vi "PeriodicFilter-Format Normal Info String.vi"(10 "Time Format String":string="%<%H:%M:%S%3u>T", 11 "Removed Info":T1[](array[typedef])) -> (3 "Array":string[](array[string]))   [LabVIEW 2017, in "Communicable State Machine.lvlib"]
uses:
  Communicable State Machine.lvlib
  Periodic String Filter Info.ctl
  _Shared/CSM Shared.lvlib
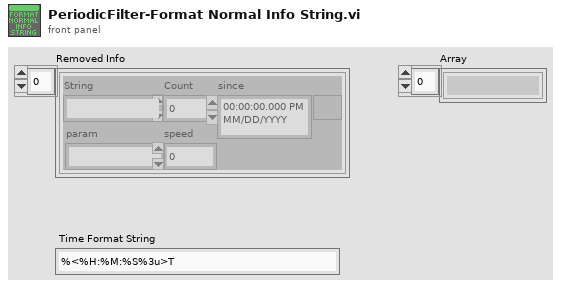
[diagram p1: front panel]
types:
  T1 = typedef "Communicable State Machine.lvlib/Periodic String Filter Info.ctl" = cluster{"String":string, "Count":i64, "since":timestamp, "param":string, "speed":dbl}
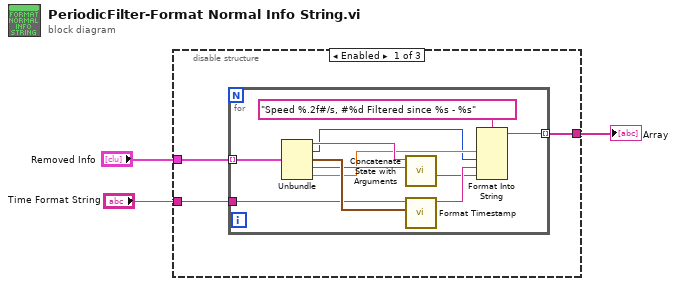
[diagram p0: block diagram]
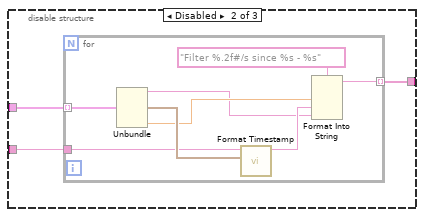
[diagram p2: hidden frame]
diagram:
  n1 = disable-structure shown="Enabled" {
    disable-tunnel: "Time Format String" -> [w6 w20 _]
    disable-tunnel: [w5 w19 _] -> w2
    disable-tunnel: "Removed Info" -> [w4 w18 _]
    frame Enabled {
      n2 = for {
        tunnel: w4 -> [w16] mode=indexing
        tunnel: [w17] -> w5 mode=indexing
        tunnel: w6 -> [w10]
        n3 = Unbundle(w16) -> ("String"=w12:string, "Count"=w7:i64, "since"=w14:timestamp, "param"=w9:string, "speed"=w8:dbl)
        n4 = call "Concatenate State with Arguments.vi"("Arguments"=w9, "State"=w12) -> ("State With Arguements"=w11:string)  [unwired: 9 in]
        n5 = call "Format Timestamp.vi"("Timestamp"=w14, "Format String"=w10) -> ("String"=w13:string)  [unwired: 9 in]
        n6 = Format Into String(format string="Speed %.2f#/s, #%d Filtered since %s - %s", w8, w7, w13, w11) -> (resulting string=w17:string)  [unwired: 2 in, 1 out]
      }
    }
    frame Disabled {
      n7 = for {
        tunnel: w18 -> [w27] mode=indexing
        tunnel: [w28] -> w19 mode=indexing
        tunnel: w20 -> [w23]
        n8 = Unbundle(w27) -> ("String"=w21:string, "since"=w25:timestamp, "speed"=w22:dbl)  [unwired: 2 out]
        n9 = call "Format Timestamp.vi"("Timestamp"=w25, "Format String"=w23) -> ("String"=w24:string)  [unwired: 9 in]
        n10 = Format Into String(format string="Filter %.2f#/s since %s - %s", w22, w24, w21) -> (resulting string=w28:string)  [unwired: 2 in, 1 out]
      }
    }
    frame Disabled {
    }
  }
  "Array" <- w2
